vi "PQ Test Invalid Connection.vi"(8 "error in (no error)":errorcluster, 10 "Connection String":string="user = llab_reader") -> (0 "error out":errorcluster)   [LabVIEW 2019]
uses:
  <vilib>/addons/_JKI Toolkits/Caraya/classes/Assert/Assert Not Error.vi
  src/LV-Data.PG/LV-Data.PGSQL.lvclass
  <vilib>/addons/_JKI Toolkits/Caraya/classes/Assert/Assert.lvclass
  <vilib>/addons/_JKI Toolkits/Caraya/classes/Test/Test.lvclass
panel:
  out "delimited string":string
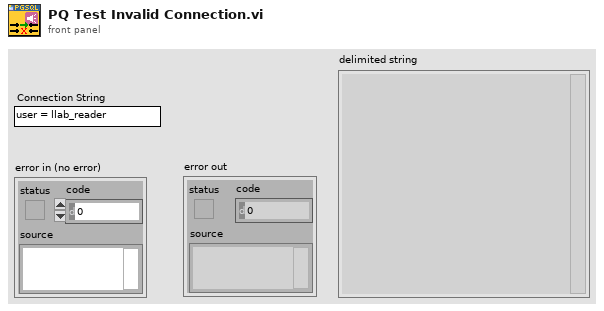
[diagram p1: front panel]
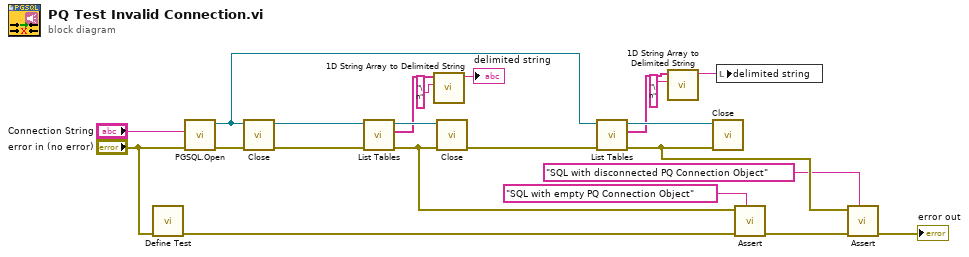
[diagram p0: block diagram]
diagram:
  n1 = call <vilib>:"Define Test.vi"("error in (no error)"="error in (no error)") -> ("error out"=w21:errorcluster)  [unwired: 9 in, 1 out]
  n2 = call "PGSQL.Open.vi"("error in (no error)"="error in (no error)", "Connection String"="Connection String") -> ("error out"=w15:errorcluster, "Data.PG out"=w11:refnum<class "LV-Data.PGSQL.lvclass">)  [unwired: 8 in]
  n3 = call-dynamic "Close.vi"("error in (no error)"=w15, "Data.PG in"=w11) -> ("error out"=w1:errorcluster, "Data.PG out"=w14:refnum<class "LV-Data.PGSQL.lvclass">)  [unwired: 8 in]
  n4 = call "List Tables.vi"("error in (no error)"=w1, "Data.PG"=w14) -> ("error out"=w12:errorcluster, "Table Names"=w19:string[], "Data.PG"=w20:refnum<class "LV-Data.PGSQL.lvclass">)  [unwired: 6 in, 1 out]
  n5 = call <vilib>:"1D String Array to Delimited String.vi"("delimiter"="\n", "string array"=w19) -> ("delimited string"=→"delimited string":string)  [unwired: 9 in]
  n6 = call-dynamic "Close.vi"("error in (no error)"=w12, "Data.PG in"=w20) -> ("error out"=w3:errorcluster)  [unwired: 8 in, 1 out]
  n7 = call "List Tables.vi"("error in (no error)"=w3, "Data.PG"=w11) -> ("error out"=w8:errorcluster, "Table Names"=w10:string[], "Data.PG"=w13:refnum<class "LV-Data.PGSQL.lvclass">)  [unwired: 6 in, 1 out]
  n8 = call <vilib>:"1D String Array to Delimited String.vi"("delimiter"="\n", "string array"=w10) -> ("delimited string"=w2:string)  [unwired: 9 in]
  n9 = call-dynamic "Close.vi"("error in (no error)"=w8, "Data.PG in"=w13) -> ()  [unwired: 8 in, 2 out]
  n10 = local write "delimited string"(w2) -> ()
  n11 = call-poly <vilib>:"Assert.vi"("Label"="SQL with empty PQ Connection Object", "error in (no error)"=w21, "Not Error?"=w12) -> ("error out"=w7:errorcluster)  [unwired: 7 in, 1 out]
  n12 = call-poly <vilib>:"Assert.vi"("Label"="SQL with disconnected PQ Connection Object", "error in (no error)"=w7, "Not Error?"=w8) -> ("error out"=→"error out":errorcluster)  [unwired: 7 in, 1 out]
